vi "Rawdata_Metadata_Analyzer.vi"() -> ()   [LabVIEW 2020]
uses:
  ctl/Image_Metadata.ctl
panel:
  out "error out":errorcluster
  out "Metadata":T1[](array[typedef]) {"Image Data Type" format="%x"}
  out "Num of Meatadata":i64
  in  "Metadata File Path":path
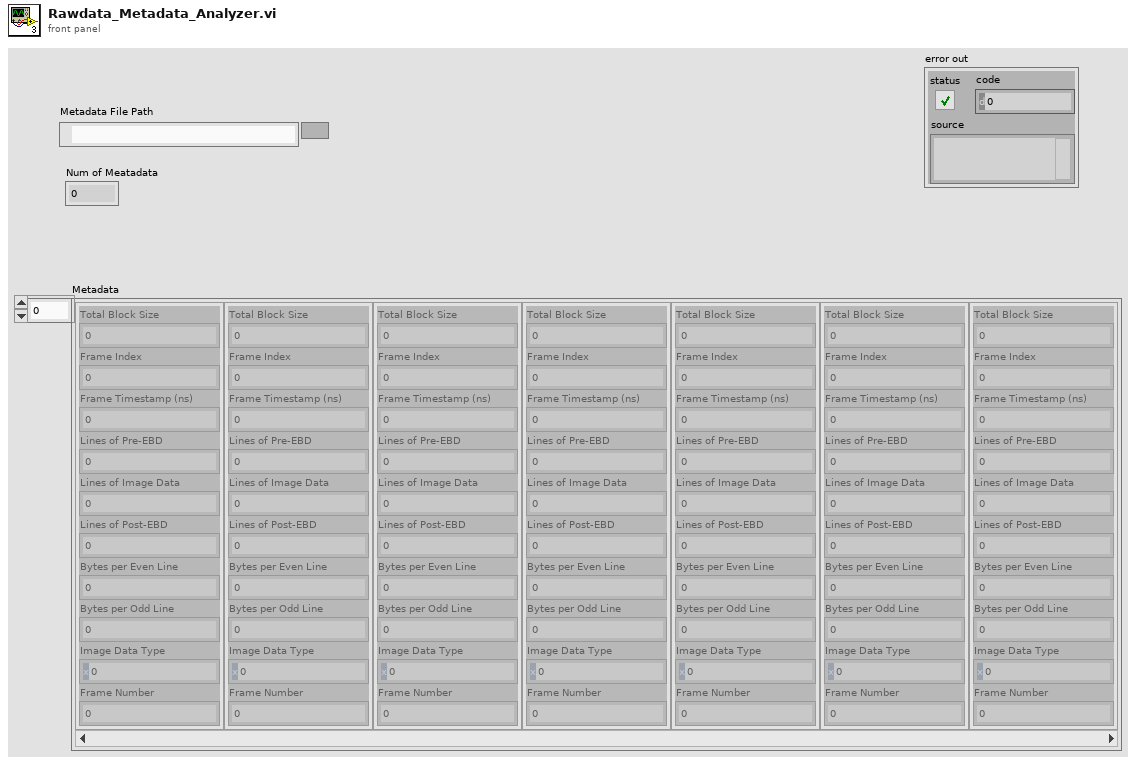
[diagram p1: front panel]
types:
  T1 = typedef "Image_Metadata.ctl" = cluster{"Total Block Size":u32, "Frame Index":u32, "Frame Timestamp (ns)":u64, "Lines of Pre-EBD":u16, "Lines of Image Data":u16, "Lines of Post-EBD":u16, "Bytes per Even Line":u16, "Bytes per Odd Line":u16, "Image Data Type":u8, "Frame Number":u16}
  T2 = enum16{"big-endian, network order", "native, host order", "little-endian"}
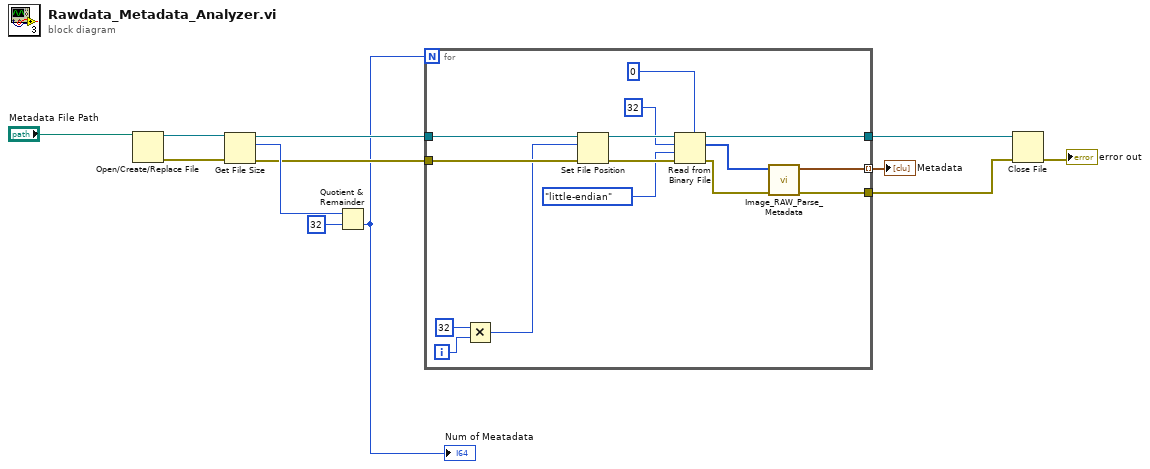
[diagram p0: block diagram]
diagram:
  n1 = Open/Create/Replace File(file path (use dialog)="Metadata File Path") -> (refnum out=w11:refnum<file>, error out=w10:errorcluster)  [unwired: 5 in, 1 out]
  n2 = Get File Size(file=w11, error in=w10) -> (refnum out=w7:refnum<file>, size (in bytes)=w9:i64, 0:w6:errorcluster)
  n3 = Quotient & Remainder(x=w9, y=i64 32) -> (floor(x/y)=w5:i64)  [unwired: 1 out]
  "Num of Meatadata" <- w5
  n4 = for {
    N: w5 -> [_]
    tunnel: w7 -> [w27]
    tunnel: w6 -> [w26]
    tunnel: [w15] -> w4 mode=indexing
    tunnel: [w14] -> w2
    tunnel: [w13] -> w3
    i -> [w25]
    n5 = Multiply(x=32, y=w25) -> (x*y=w23:i32)
    n6 = Set File Position(offset (in bytes) (0)=w23, refnum=w27, error in=w26) -> (refnum out=w22:refnum<file>, error out=w21:errorcluster)  [unwired: 1 in]
    n7 = Read from Binary File(5:u8 0, 8:w21, 9:T2."little-endian" ("byte order (0:big-endian, network order)"), 10:32 ("count (1)"), 11:w22) -> (0:w17:errorcluster, 2:w16:u8[], 3:w13:refnum<file>)  [unwired: 1 in, 1 out]
    n8 = call "Image_RAW_Parse_Metadata.vi"("error in (no error)"=w17, "Metadata (U8)"=w16) -> ("error out"=w14:errorcluster, "Image Metadata"=w15:T1)  [unwired: 8 in]
  }
  "Metadata" <- w4
  n9 = Close File(refnum=w3, error in=w2) -> (error out=→"error out":errorcluster)  [unwired: 1 out]
